vi "Create Observer.vi"(8 "error in (no error)":errorcluster) -> (0 "error out":errorcluster, 3 "System Config":refnum<event-registration>)   [LabVIEW 2015, in "System Config.lvclass"]
uses:
  System Config.lvclass
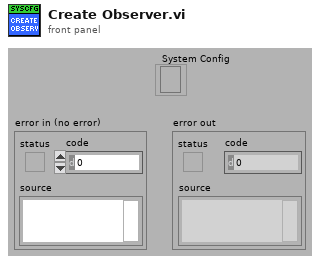
[diagram p1: front panel]
types:
  T1 = typedef "System Config.lvclass/ClassAttributes.ctl" = cluster{"Config":cluster{"Logging":cluster{"Log Files Directory":path, "Max Lines Per Log File":i32}, "Settings":T2}, "Core":cluster{"Config Directory":path, "Name":string, "Config Changed":refnum<user-event>}}
  T2 = typedef "System Config.lvclass/Settings.ctl" = cluster{"Dummy":dbl}
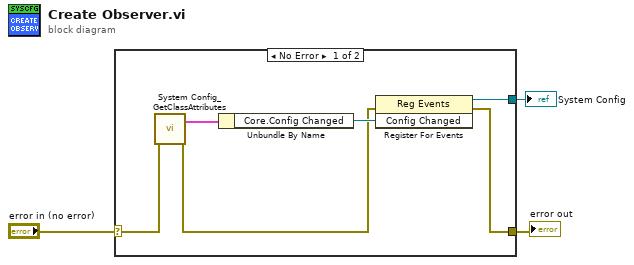
[diagram p0: block diagram]
diagram:
  n1 = case shown="No Error" "error in (no error)" {
    selector: "error in (no error)" -> [w9 w10]
    tunnel: [w4 w10] -> w2
    tunnel: [w6 _] -> w1
    frame No Error {
      n2 = call "System Config_GetClassAttributes.vi"("error in (no error)"=w9) -> ("error out"=w5:errorcluster, "class attributes"=w8:T1)  [unwired: 7 in, 2 out]
      n3 = Unbundle By Name(w8) -> ("Core.Config Changed"=w7:refnum<user-event>)
      n4 = register-events(error in=w5, w7) -> (reference out=w6:refnum<event-registration>, error out=w4:errorcluster)  [unwired: 1 in]
    }
    frame Error {
    }
  }
  "error out" <- w2
  "System Config" <- w1
